vi "get_timestamp_from_distance.vi"(8 "distance":dbl=1000.0, 9 "manual end":timestamp, 10 "start":timestamp, 11 "lat/lon position":T1) -> (0 "time between timestamps":dbl, 1 "distance":dbl, 2 "mean speed":dbl, 3 "end time":timestamp)   [LabVIEW 2020]
uses:
  <vilib>/Analysis/1siggen.llb/Ramp Pattern by Delta.vi
  <vilib>/Analysis/NI_AALBase.lvlib
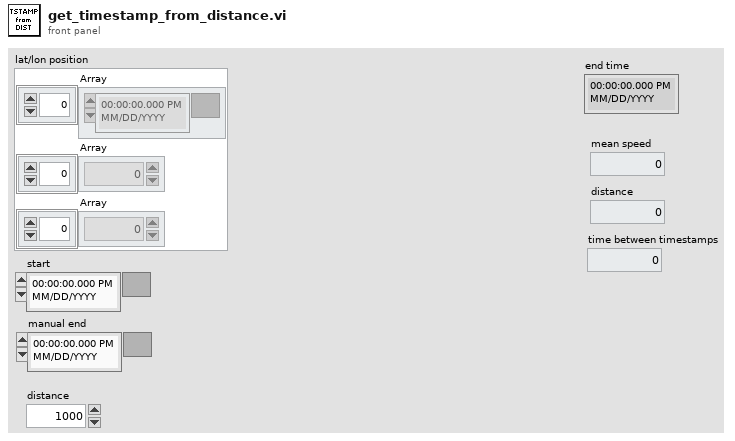
[diagram p1: front panel]
types:
  T1 = cluster{"Array":timestamp[], "Array":dbl[], "Array":dbl[]}
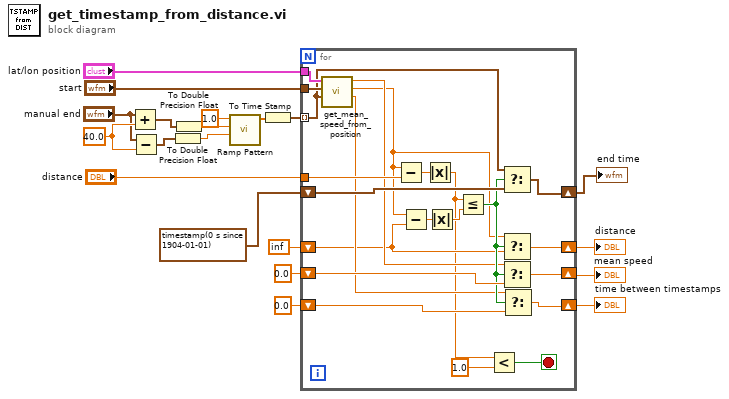
[diagram p0: block diagram]
diagram:
  w13 = 40.0 ("delta")
  n1 = Add(x="manual end", y=w13) -> (x+y=w15:timestamp)
  n2 = Subtract(x="manual end", y=w13) -> (x-y=w16:timestamp)
  n3 = To Double Precision Float(number=w16) -> (double precision float=w17:dbl)
  n4 = To Double Precision Float(number=w15) -> (double precision float=w14:dbl)
  n5 = call-poly <vilib>:"Ramp Pattern.vi"("start"=w17, "end"=w14, "delta"=1.0) -> ("Ramp Pattern"=w18:dbl[])  [unwired: 6 in, 2 out]
  n6 = To Time Stamp(1:w18) -> (0:w19:timestamp[])
  n7 = for {
    tunnel: "start" -> [w38]
    tunnel: "lat/lon position" -> [w42]
    tunnel: w19 -> [w21] mode=indexing
    tunnel: "distance" -> [w40]
    shift-right: [w39] -> w7
    shift-left: inf -> [w26]
    shift-right: [w35] -> w5
    shift-left: 0.0 ("mean speed [m/s]") -> [w34]
    shift-right: [w31] -> w6
    shift-left: 0.0 ("dt [s]") -> [w32]
    shift-right: [w36] -> w4
    shift-left: timestamp(0 s since 1904-01-01) ("start") -> [w37]
    stop <- w24 stop-if-true
    n8 = call "get_mean_speed_from_position.vi"("end"=w21, "start"=w38, "lat/lon position"=w42) -> ("dt [s]"=w29:dbl, "distance [m]"=w25:dbl, "mean speed [m/s]"=w30:dbl)  [unwired: 6 in]
    n9 = Subtract(x=w25, y=w40) -> (x-y=w41:dbl)
    n10 = Subtract(x=w25, y=w26) -> (x-y=w28:dbl)
    n11 = Absolute Value(x=w41) -> (abs(x)=w22:dbl)
    n12 = Absolute Value(x=w28) -> (abs(x)=w27:dbl)
    n13 = Less Or Equal?(x=w22, y=w27) -> (x <= y?=w33:bool)
    n14 = Less?(x=w22, y=1.0) -> (x < y?=w24:bool)
    n15 = Select(t=w21, s=w33, f=w37) -> (s? t:f=w36:timestamp)
    n16 = Select(t=w25, s=w33, f=w26) -> (s? t:f=w39:dbl)
    n17 = Select(t=w30, s=w33, f=w34) -> (s? t:f=w35:dbl)
    n18 = Select(t=w29, s=w33, f=w32) -> (s? t:f=w31:dbl)
  }
  "distance" <- w7
  "mean speed" <- w5
  "time between timestamps" <- w6
  "end time" <- w4
